vi "Bundle.vi"(8 "error in (no error)":errorcluster, 9 "Request ID":u32, 10 "Data":refnum<class "Data.lvclass">, 11 "Request Data in":refnum<class "Request Data.lvclass">) -> (0 "error out":errorcluster, 3 "Request Data out":refnum<class "Request Data.lvclass">)   [LabVIEW 2020, in "Publisher.lvlib" / "Request Data.lvclass"]
doc: "Write Data and Request ID to the Request Data."
uses:
  Request Data.lvclass
  PPL/HDH.Data.Generic.lvlibp/Data.lvclass
  Request Data.lvclass/Request Data.ctl
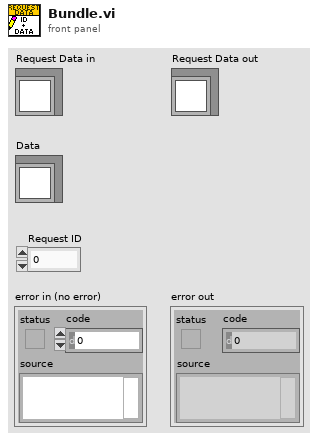
[diagram p1: front panel]
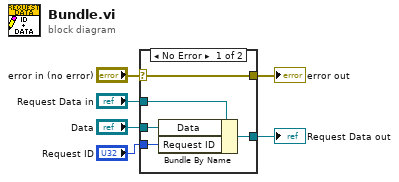
[diagram p0: block diagram]
diagram:
  n1 = case shown="No Error" "error in (no error)" {
    selector: "error in (no error)" -> [w11 w12]
    tunnel: [w11 w12] -> w5
    tunnel: [w9 w13] -> w3
    tunnel: "Request Data in" -> [w10 w13]
    tunnel: "Data" -> [w8 _]
    tunnel: "Request ID" -> [w7 _]
    frame No Error {
      n2 = Bundle By Name(cluster=w10, "Data"=w8, "Request ID"=w7) -> (w9:refnum<class "Request Data.lvclass">)
    }
    frame Error {
    }
  }
  "error out" <- w5
  "Request Data out" <- w3
